vi "Headers.vi"() -> (3 "Headers":string[](array[string]))   [LabVIEW 2013]
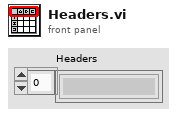
[diagram p1: front panel]
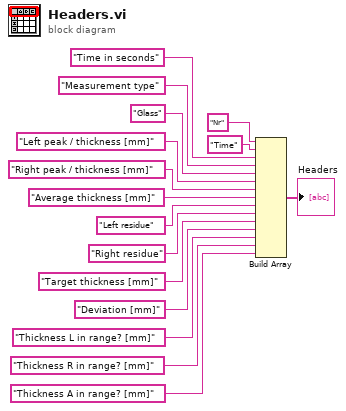
[diagram p0: block diagram]
diagram:
  n1 = Build Array("Nr" ("element"), "Time" ("element"), "Time in seconds" ("element"), "Measurement type" ("element"), "Glass" ("element"), "Left peak / thickness [mm]", "Right peak / thickness [mm]", "Average thickness [mm]", "Left residue", "Right residue", "Target thickness [mm]" ("element"), "Deviation [mm]" ("element"), "Thickness L in range? [mm]", "Thickness R in range? [mm]", "Thickness A in range? [mm]") -> (→"Headers":string[])
